vi "OE1022D_Configure Auto Setting.vi"(7 "OE1022D_Auto Setting":T1={"Auto Gain"=FALSE, "Auto Reserve"=FALSE, "Auto Phase"=FALSE, "Auto Scale"=FALSE, "Channel"=1} {"Channel" items=["A"=1, "B"=2]}, 8 "Error in (no error)":errorcluster caption="error out（no error）", 9 "Remote Mode":u16(ring) items=["USB", "RS232", "GPIB"], 11 "VISA resource name":refnum<visa-resource-name>) -> (0 "Error out":errorcluster caption="error out", 1 "Output String":string, 3 "VISA resource  out":refnum<visa-resource-name>)   [LabVIEW 2019]
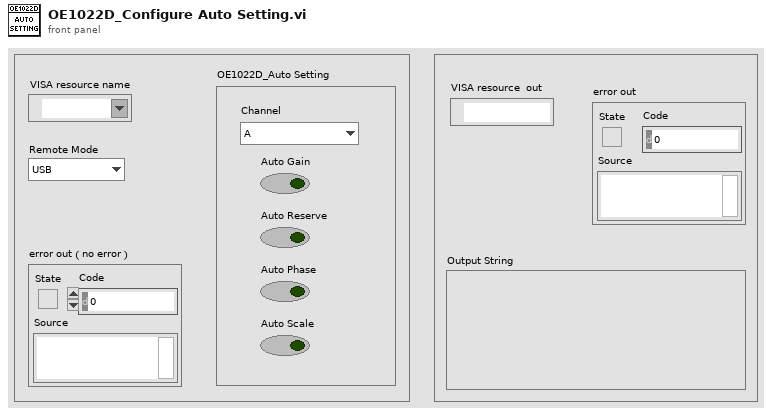
[diagram p1: front panel]
types:
  T1 = cluster{"Auto Gain":bool, "Auto Reserve":bool, "Auto Phase":bool, "Auto Scale":bool, "Channel":u16}
  T2 = enum16{"ISRC", "IGND", "ICPL", "ILIN", "PHAS", "FMOD", "RSLP", "FREQ", "SWPT", "SLLM", "SULM", "SSLL", "SSLG", "STLM", "SWRM", "IRNG", "SENS", "RMOD", "OFLT", "OFSL", "SYNC", "DMOD", "HARM", "DARB", "SWVT", "SLVL", "SVLL", "SVUL", "SVSL", "SVSG", "SVTM", "SVRM", "RALL", "SNAP", "OUTP", "OAUX", "COUT", "CAUX", "COFP", "CEXP", "FPOP", "OEXP", "*IDN", "*RST", "OVLD", "INOV", "GNOV", "*PLL", "SSET", "RSET", "AGAN", "APHS", "ARSV", "ASCL", "EQCD", "EQCS", "SPED", "SRAT", "SLEN", "SSLE", "STRG", "SPRM", "STRD", "PAUS", "REST", "SPTS", "TRCA", "TEMP", "RSTU", "IHNZ", "DEQU", "SADD", "ARNG", "CSPE", "ISRCD", "IGNDD", "ICPLD", "ILIND", "PHASD", "FMODD", "RSLPD", "FREQD", "SWPTD", "SLLMD", "SULMD", "SSLLD", "SSLGD", "STLMD", "SWRMD", "SENSD", "RMODD", "OFLTD", "OFSLD", "SYNCD", "HARMD", "EQCDD", "EQCSD", "SNAPD", "OUTPD", "SWVTD", "SLVLD", "SVLLD", "SVULD", "SVSLD", "SVSGD", "SVTMD", "SVRMD", "SVDCD", "ARSVD", "AGAND", "APHSD", "ASCLD", "FPOPD", "CAUXD", "OEXPD", "SPEDD", "SRATD", "SLEND", "SSLED", "STRGD", "SPRMD", "STRDD", "PAUSD", "RESTD", "SPTSD", "TRCAD", "*IDND", "*RSTD", "INOVD", "GNOVD", "*PLLD", "SSETD", "RSETD"}
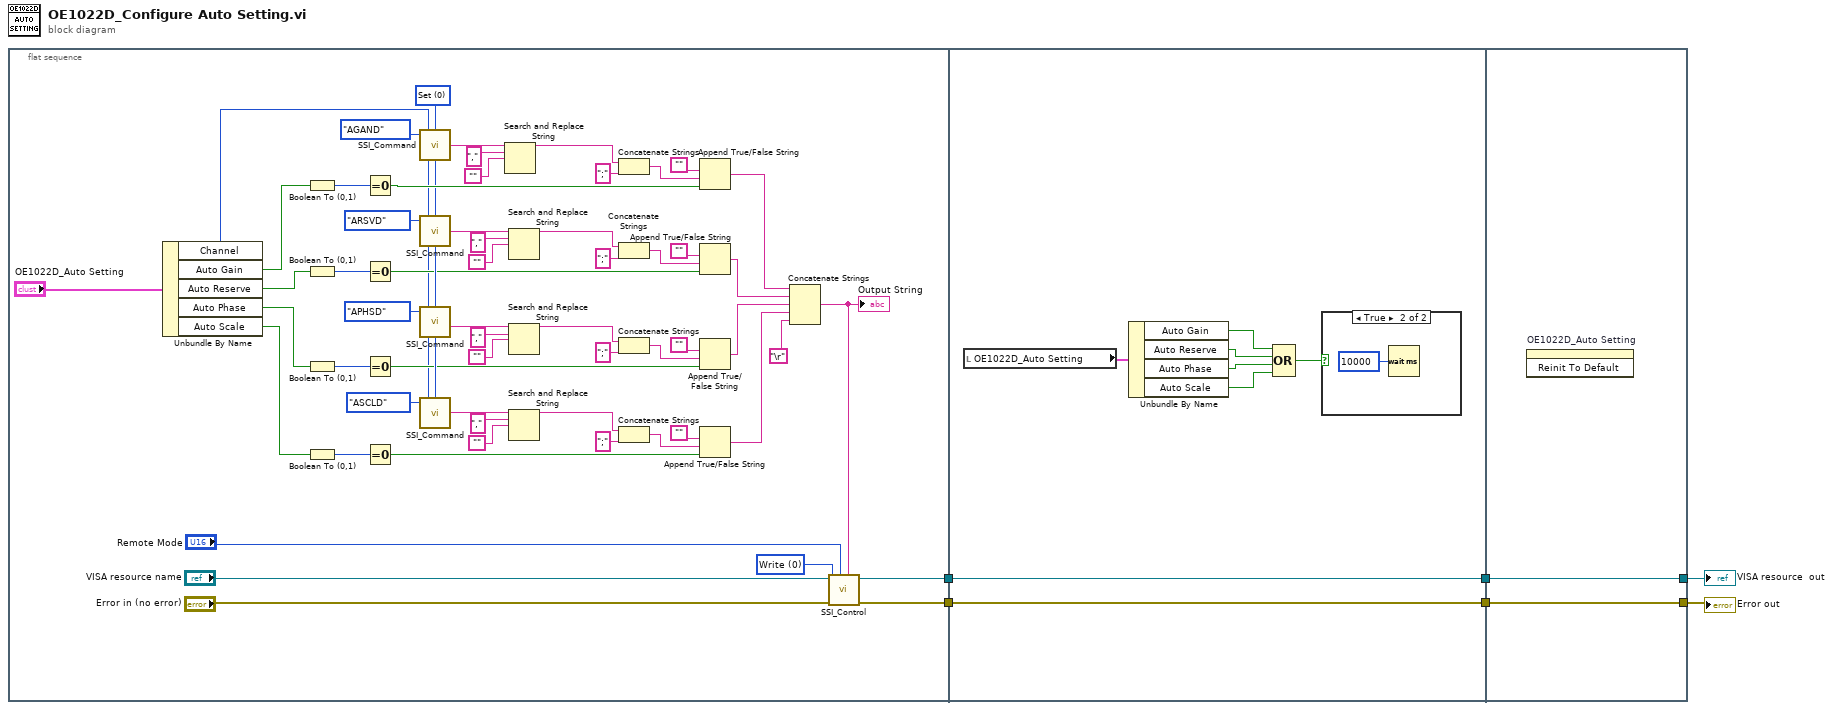
[diagram p0: block diagram]
diagram:
  n1 = flat-sequence {
    tunnel: [w38] -> w6
    tunnel: [w37] -> w5
    tunnel: w6 -> [w73]
    tunnel: w5 -> [w72]
    tunnel: [w73] -> w2
    tunnel: [w72] -> w1
    tunnel: [w75] -> w4
    tunnel: [w76] -> w3
    tunnel: w2 -> [w76]
    tunnel: w1 -> [w75]
    frame #0 {
      w42 = u16 0 items=["Write", "Read"] ("Control")
      w61 = u16 0 items=["Set", "Query"] ("Opera")
      n2 = Unbundle By Name("OE1022D_Auto Setting") -> ("Channel"=w35:u16, "Auto Gain"=w64:bool, "Auto Reserve"=w50:bool, "Auto Phase"=w49:bool, "Auto Scale"=w48:bool)
      n3 = Boolean To (0,1)(Boolean=w64) -> (0, 1=w62:i16)
      n4 = Boolean To (0,1)(Boolean=w50) -> (0, 1=w58:i16)
      n5 = Boolean To (0,1)(Boolean=w49) -> (0, 1=w54:i16)
      n6 = Boolean To (0,1)(Boolean=w48) -> (0, 1=w52:i16)
      n7 = Equal To 0?(x=w62) -> (x = 0?=w63:bool)
      n8 = Equal To 0?(x=w58) -> (x = 0?=w59:bool)
      n9 = Equal To 0?(x=w54) -> (x = 0?=w53:bool)
      n10 = Equal To 0?(x=w52) -> (x = 0?=w51:bool)
      n11 = call "SSI_Command.vi"("Opera"=w61, "channel"=w35, "Command Type"=T2."AGAND") -> ("Output string"=w22:string)  [unwired: 1 in]
      n12 = call "SSI_Command.vi"("Opera"=w61, "channel"=w35, "Command Type"=T2."ARSVD") -> ("Output string"=w17:string)  [unwired: 1 in]
      n13 = call "SSI_Command.vi"("Opera"=w61, "channel"=w35, "Command Type"=T2."APHSD") -> ("Output string"=w13:string)  [unwired: 1 in]
      n14 = call "SSI_Command.vi"("Opera"=w61, "channel"=w35, "Command Type"=T2."ASCLD") -> ("Output string"=w9:string)  [unwired: 1 in]
      n15 = Search and Replace String(input string=w22, search string="," ("搜索字符串"), replace string="") -> (result string=w19:string)  [unwired: 5 in, 3 out]
      n16 = Search and Replace String(input string=w17, search string="," ("搜索字符串"), replace string="") -> (result string=w15:string)  [unwired: 5 in, 3 out]
      n17 = Search and Replace String(input string=w13, search string="," ("搜索字符串"), replace string="") -> (result string=w11:string)  [unwired: 5 in, 3 out]
      n18 = Search and Replace String(input string=w9, search string="," ("搜索字符串"), replace string="") -> (result string=w7:string)  [unwired: 5 in, 3 out]
      n19 = Concatenate Strings(w19, ";") -> (w30:string)
      n20 = Concatenate Strings(w15, ";") -> (w29:string)
      n21 = Concatenate Strings(w11, ";") -> (w28:string)
      n22 = Concatenate Strings(w7, ";") -> (w27:string)
      n23 = Append True/False String(1:w63, 2:w30, 3:"") -> (0:w26:string)  [unwired: 1 in]
      n24 = Append True/False String(1:w59, 2:w29, 3:"") -> (0:w25:string)  [unwired: 1 in]
      n25 = Append True/False String(1:w53, 2:w28, 3:"") -> (0:w23:string)  [unwired: 1 in]
      n26 = Append True/False String(1:w51, 2:w27, 3:"") -> (0:w24:string)  [unwired: 1 in]
      n27 = Concatenate Strings(w26, w25, w23, w24, "\r") -> (w39:string)
      "Output String" <- w39
      n28 = call "SSI_Control.vi"("Write Buffer"=w39, "Remote Mode"="Remote Mode", "Error in (no error)"="Error in (no error)", "Control"=w42, "VISA resource name"="VISA resource name") -> ("Error out"=w37:errorcluster, "VISA resource  out"=w38:refnum<visa-resource-name>)  [unwired: 3 in, 2 out]
    }
    frame #1 {
      n29 = local read "OE1022D_Auto Setting"() -> (w71:T1)
      n30 = Unbundle By Name(w71) -> ("Auto Gain"=w67:bool, "Auto Reserve"=w68:bool, "Auto Phase"=w69:bool, "Auto Scale"=w70:bool)
      n31 = Compound Arithmetic op=OR(w67, w68, w69, w70) -> (w66:bool)
      n32 = case shown="True" w66 {
        frame False {
        }
        frame True {
          n33 = Wait (ms)(milliseconds to wait=u32 10000 ("等待时间（毫秒）")) -> ()  [unwired: 1 out]
        }
      }
    }
    frame #2 {
      n34 = invoke on="OE1022D_Auto Setting" class="Clust (严格)" method="Reinit To Default"() -> ()  [unwired: 3 in, 3 out]
    }
  }
  "Error out" <- w4
  "VISA resource  out" <- w3
